vi "Get Invalid Scalar Data Channels.vi"(8 "error in (no error)":errorcluster, 10 "new bitfile scalar channels":T1[](array[typedef]) {"Data Type" format="%.0x"}, 11 "old bitfile scalar channels":T1[](array[typedef]) {"Data Type" format="%.0x"}) -> (0 "error out":errorcluster, 2 "still valid data channels":T1[](array[typedef]) {"Data Type" format="%.0x"}, 3 "invalid scalar data channels":T1[](array[typedef]) {"Data Type" format="%.0x"})   [LabVIEW 2018]
uses:
  Addon Shared/Types/Register Information.ctl
  Addon Shared/Types/Data Type.ctl
  Addon Shared/FPGA Addon Shared.lvlib
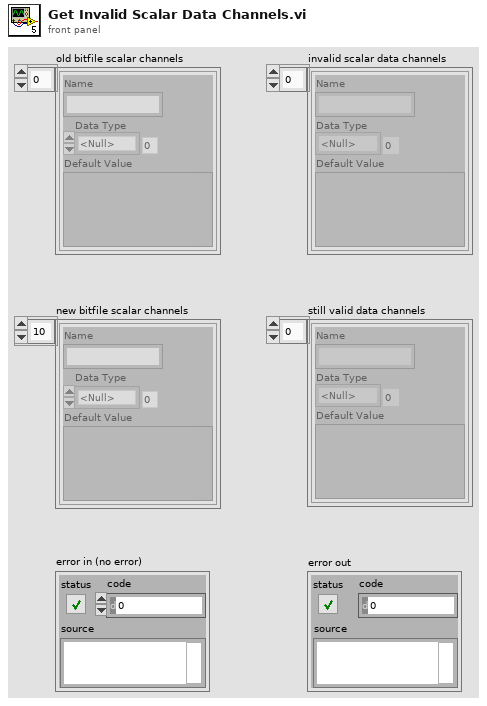
[diagram p1: front panel]
types:
  T1 = typedef "FPGA Addon Shared.lvlib/Register Information.ctl" = cluster{"Name":string, "Data Type":T2, "Default Value":variant}
  T2 = typedef "FPGA Addon Shared.lvlib/Data Type.ctl" = enum8{"<Null>", "I8", "I16", "I32", "I64", "U8", "U16", "U32", "U64", "SGL", "Boolean", "Analog PWM In Settings", "Analog PWM In", "Digital PWM In Settings", "Digital PWM In", "Digital PWM Out", "Sine Out", "FXP+/-24.5", "FXP+/-16.5", "FXP+/-32.8", "FXP+/-64.32", "FXP+/-16.7", "FXP+/-20.5", "FXP+/-27.5", "FXP+/-32.16", "FXP+16.3", "FXP+18.3", "Digital Static In", "Digital Static Out", "Digital Static In Settings", "Digital WSS Out", "Quad Encoder Settings", "Quad Encoder In", "Group"}
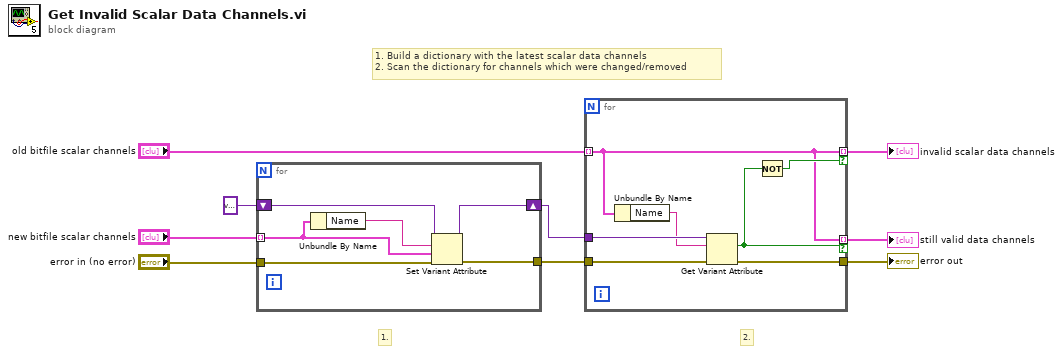
[diagram p0: block diagram]
diagram:
  # "1. Build a dictionary with the latest scalar data channels\n2. Scan the dictionary for channels which were changed/removed"
  # "2."
  # "1."
  n1 = for {
    tunnel: "new bitfile scalar channels" -> [w12] mode=indexing
    tunnel: "error in (no error)" -> [w14]
    tunnel: [w13] -> w7
    shift-right: [w10] -> w9
    shift-left: variant -> [w11]
    n2 = Unbundle By Name(w12) -> ("Name"=w15:string)
    n3 = Set Variant Attribute(Variant=w11, name=w15, value=w12, error in=w14) -> (Variant out=w10:variant, error out=w13:errorcluster)  [unwired: 1 out]
  }
  n4 = for {
    tunnel: [w21] -> w8
    tunnel: w7 -> [w22]
    tunnel: w9 -> [w20]
    tunnel: "old bitfile scalar channels" -> [w17] mode=indexing
    tunnel: [w17] -> w3 mode=indexing if=w18
    tunnel: [w17] -> w2 mode=indexing if=w16
    n5 = Unbundle By Name(w17) -> ("Name"=w19:string)
    n6 = Get Variant Attribute(Variant=w20, name=w19, error in=w22) -> (found=w16:bool, error out=w21:errorcluster)  [unwired: 1 in, 2 out]
    n7 = Not(x=w16) -> (.not. x?=w18:bool)
  }
  "error out" <- w8
  "invalid scalar data channels" <- w3
  "still valid data channels" <- w2
